vi "TWM Client Cmd Set Multiplexer Paths.vi"(5 "timeout [ms]":i32=5000, 7 "end of packet key":string="TWM:command:EndOfPacket", 8 "error in":errorcluster, 10 "mux paths":T1[](array[typedef]), 11 "handle":i32) -> (0 "error out":errorcluster, 3 "handle out":i32)   [LabVIEW 2020, in "TWM Client.lvlib"]
doc: "This will define multiplexer paths. It is equivalent to manual definition of paths (channels) in multiplexer panel. It works only for generic multiplexers (some of them). Otherwise it do nothing."
uses:
  TWM Client.lvlib
  octave/infolib/infolib.lvlib
  octave/infolib/1D String.vi
  TWM Client Mux Path.ctl
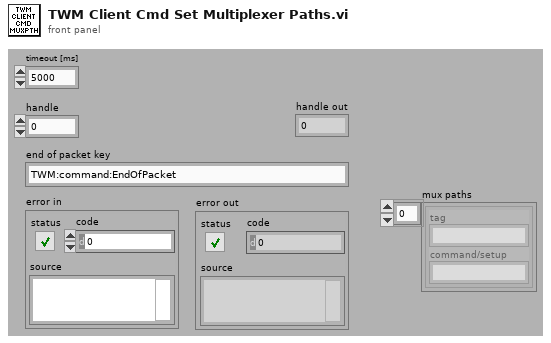
[diagram p1: front panel]
types:
  T1 = typedef "TWM Client.lvlib/TWM Client Mux Path.ctl" = cluster{"tag":string, "command/setup":string}
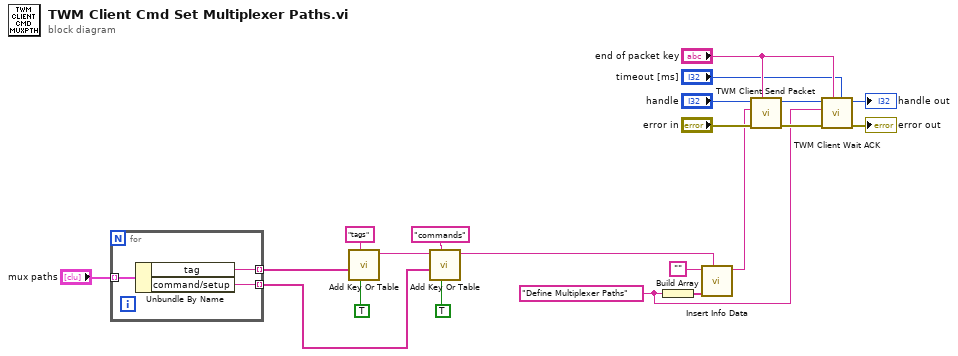
[diagram p0: block diagram]
diagram:
  w12 = "Define Multiplexer Paths" ("section name")
  n1 = for {
    tunnel: "mux paths" -> [w24] mode=indexing
    tunnel: [w23] -> w8 mode=indexing
    tunnel: [w22] -> w2 mode=indexing
    n2 = Unbundle By Name(w24) -> ("tag"=w23:string, "command/setup"=w22:string)
  }
  n3 = call-poly "Add Key Or Table.vi"("collumn vector (F)"=TRUE, "key description"="tags", "string"=w8) -> ("info data out"=w3:string)  [unwired: 7 in, 1 out]
  n4 = call-poly "Add Key Or Table.vi"("collumn vector (F)"=TRUE, "key description"="commands", "string"=w2, "info data"=w3) -> ("info data out"=w1:string)  [unwired: 6 in, 1 out]
  n5 = Build Array(w12) -> (w18:string[])
  n6 = call "Insert Info Data.vi"("info data to insert"=w1, "sections"=w18, "info data"="") -> ("info data out"=w19:string)  [unwired: 7 in, 1 out]
  n7 = call "TWM Client Send Packet.vi"("end of packet key"="end of packet key", "error in"="error in", "command string"=w19, "handle"="handle") -> ("error out"=w14:errorcluster, "handle out"=w11:i32)  [unwired: 6 in]
  n8 = call "TWM Client Wait ACK.vi"("timeout [ms] (3000)"="timeout [ms]", "key string"="end of packet key", "error in"=w14, "command header"=w12, "handle"=w11) -> ("error out"=→"error out":errorcluster, "handle out"=→"handle out":i32)  [unwired: 5 in]
